vi "Get Selected XNET Channels.vi"(8 "error in (no error)":errorcluster, 9 "Node Ptr":u64 format="%.0x", 10 "XNET Cluster":refnum<k21>, 11 "Tree In":refnum<vi>) -> (0 "error out":errorcluster, 2 "XNET Signal Names":refnum<k21>[](array[refnum]), 3 "Tree Out":refnum<vi>)   [LabVIEW 2013, in "J1939 Addon System Explorer.lvlib"]
uses:
  J1939 Addon System Explorer.lvlib
  <resource>/objmgr/xnet.rc
  <vilib>/NI Veristand/Custom Device API/Custom Device API.lvlib
panel:
  # "OUTPUTS"
  # "INPUTS"
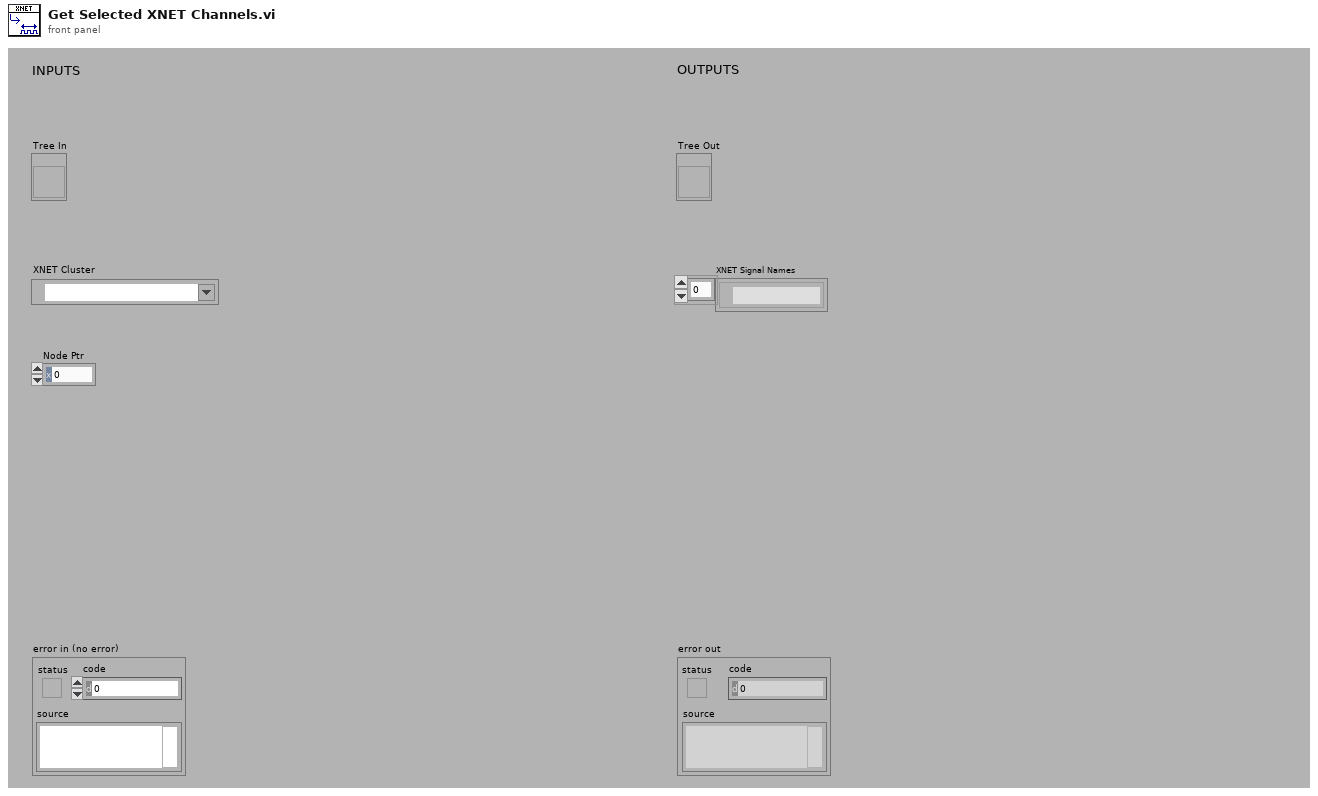
[diagram p1: front panel]
types:
  T1 = typedef "Custom Device API.lvlib/Custom Device Item Ref.ctl" = u64
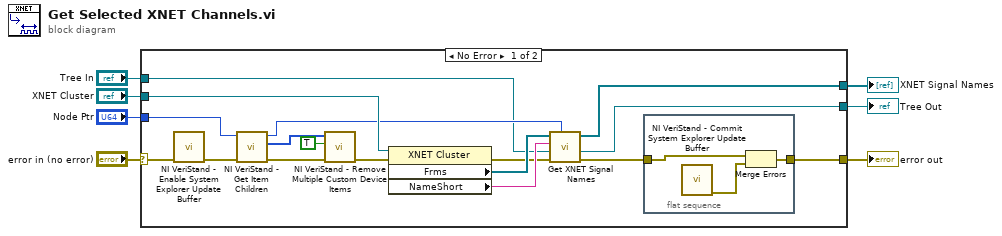
[diagram p0: block diagram]
diagram:
  n1 = case shown="No Error" "error in (no error)" {
    selector: "error in (no error)" -> [w11 w29]
    tunnel: [w8 w29] -> w6
    tunnel: "XNET Cluster" -> [w24 _]
    tunnel: [w14 _] -> w4
    tunnel: "Tree In" -> [w12 w28]
    tunnel: [w21 w28] -> w2
    tunnel: "Node Ptr" -> [w20 _]
    frame No Error {
      n2 = call <vilib>:"NI VeriStand - Enable System Explorer Update Buffer.vi"("error in (no error)"=w11) -> ("error out"=w10:errorcluster)  [unwired: 10 in]
      n3 = call <vilib>:"NI VeriStand - Get Item Children.vi"("error in (no error)"=w10, "Item Ref in"=w20) -> ("error out"=w17:errorcluster, "Child Refs"=w18:T1[], "Item Ref out"=w13:T1)  [unwired: 6 in, 1 out]
      n4 = call <vilib>:"NI VeriStand - Remove Multiple Custom Device Items.vi"("error in (no error)"=w17, "Force Delete (F)"=TRUE, "Item Refs in"=w18) -> ("error out"=w16:errorcluster)  [unwired: 7 in, 1 out]
      n5 = property class="XNET Cluster"(reference=w24, error in=w16) -> (error out=w15:errorcluster, "Frms"=w23:refnum<k21>[], "NameShort"=w22:string)  [unwired: 1 out]
      n6 = call "Get XNET Signal Names.vi"("Parent Ref in"=w13, "error in"=w15, "Tree In"=w12, "Parent"=w22, "Frms"=w23) -> ("error out"=w9:errorcluster, "Tree Out"=w21:refnum<vi>, "XNET Signal Names"=w14:refnum<k21>[])  [unwired: 4 in]
      n7 = flat-sequence {
        tunnel: w9 -> [w26]
        tunnel: [w25] -> w8
        frame #0 {
          n8 = call <vilib>:"NI VeriStand - Commit System Explorer Update Buffer.vi"() -> ("error out"=w27:errorcluster)  [unwired: 11 in]
          n9 = Merge Errors(w26, w27) -> (w25:errorcluster)
        }
      }
    }
    frame Error {
    }
  }
  "error out" <- w6
  "XNET Signal Names" <- w4
  "Tree Out" <- w2
